vi "Cmd.ReadMode.vi"(6 "Timeout [ms] (1000)":i32=1000, 8 "error in":errorcluster, 11 "cID in":refnum<k5>) -> (0 "error out":errorcluster, 2 "RunMode":T1, 3 "cID out":refnum<k5>)   [LabVIEW 2016]
uses:
  controls/RunMode.ctl
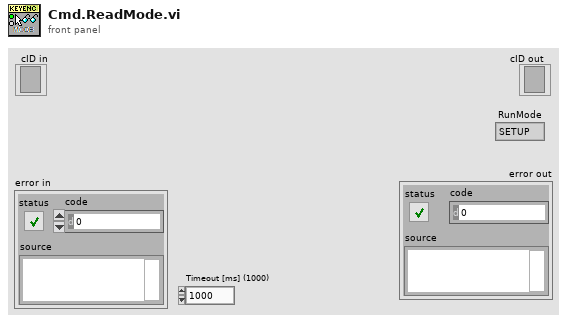
[diagram p1: front panel]
types:
  T1 = typedef "RunMode.ctl" = enum16{"SETUP", "RUN"}
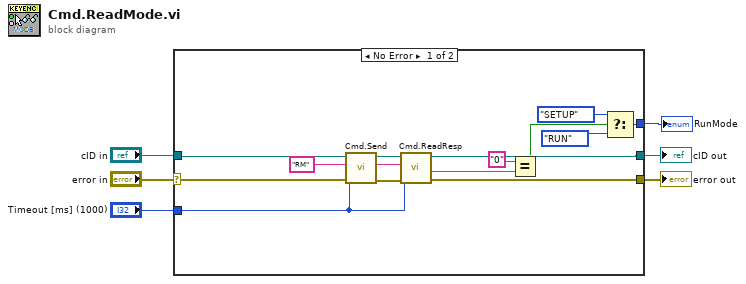
[diagram p0: block diagram]
diagram:
  n1 = case shown="No Error" "error in" {
    selector: "error in" -> [w19 w21]
    tunnel: "Timeout [ms] (1000)" -> [w16 _]
    tunnel: "cID in" -> [w20 w22]
    tunnel: [w15 w22] -> w3
    tunnel: [w14 w21] -> w2
    tunnel: [w9 _] -> w1
    frame No Error {
      w13 = "RM"
      n2 = call "Cmd.Send.vi"("error in (no error)"=w19, "Timeout [ms] (1000)"=w16, "Command"=w13, "connection ID"=w20) -> ("error out"=w17:errorcluster, "connection ID out"=w18:refnum<k5>)  [unwired: 6 in]
      n3 = call "Cmd.ReadResp.vi"("error in (no error)"=w17, "Timeout [ms] (1000)"=w16, "Request"=w13, "connection ID"=w18) -> ("error out"=w14:errorcluster, "ResponseParameters"=w7:string, "connection ID out"=w15:refnum<k5>)  [unwired: 5 in]
      n4 = Equal?(x="0", y=w7) -> (x = y?=w12:bool)
      n5 = Select(t=RunMode."SETUP" ("RunMode"), s=w12, f=RunMode."RUN" ("RunMode")) -> (s? t:f=w9:T1)
    }
    frame Error {
    }
  }
  "cID out" <- w3
  "error out" <- w2
  "RunMode" <- w1
